vi "QMH_create.vi"(8 "error in (no error)":errorcluster) -> (0 "error out":errorcluster)   [LabVIEW 2021, in "Framework_lib.lvlib"]
uses:
  Framework_lib.lvlib
  framework_Qmessage.ctl
  QMH_notifier_payload.ctl
  QMH_producer_enum.ctl
  QMH_references.ctl
  QMH_references_enum.ctl
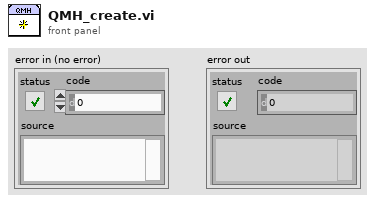
[diagram p1: front panel]
types:
  T1 = typedef "Framework_lib.lvlib/QMH_references_enum.ctl" = enum16{"--select Ref--", "Consumer_SUT", "Consumer_Annot", "Compute_Results"}
  T2 = typedef "Framework_lib.lvlib/QMH_references.ctl" = cluster{"Consumer_SUT":refnum<queue>, "Consumer_annotation":refnum<queue>, "compute_results":refnum<queue>, "Notifier":refnum<notifier>}
  T3 = typedef "Framework_lib.lvlib/QMH_notifier_payload.ctl" = cluster{"Message":T4, "Payload":variant}
  T4 = typedef "Framework_lib.lvlib/QMH_producer_enum.ctl" = enum16{"Idle", "Initialize", "Shutdown", "ERROR", "Stop", "Start", "Enqueue_frames"}
  T5 = typedef "Framework_lib.lvlib/framework_Qmessage.ctl" = cluster{"Message":string, "Payload":variant}
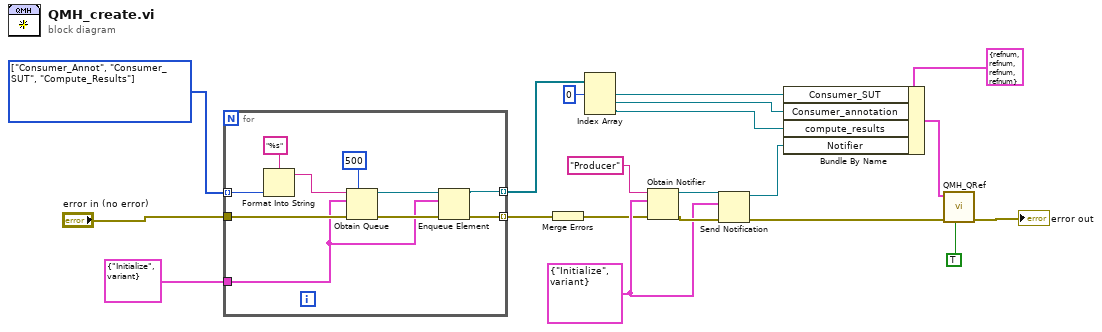
[diagram p0: block diagram]
diagram:
  w1 = T1[] [enum."Consumer_Annot", enum."Consumer_SUT", enum."Compute_Results"] items=["--select Ref--", "Consumer_SUT", "Consumer_Annot", "Compute_Results"] ("Array")
  w16 = T3 {"Message"=enum."Initialize", "Payload"=variant}
  n1 = for {
    tunnel: "error in (no error)" -> [w30]
    tunnel: w1 -> [w23] mode=indexing
    tunnel: T5 {"Message"="Initialize", "Payload"=variant} -> [w26]
    tunnel: [w25] -> w10 mode=indexing
    tunnel: [w24] -> w8 mode=indexing
    n2 = Format Into String(format string="%s", w23) -> (resulting string=w21:string)  [unwired: 2 in, 1 out]
    n3 = Obtain Queue(max queue size (-1, unlimited)=500, name (unnamed)=w21, element data type=w26, error in (no error)=w30) -> (queue out=w28:refnum<queue>, error out=w29:errorcluster)  [unwired: 1 in, 1 out]
    n4 = Enqueue Element(queue=w28, element=w26, error in (no error)=w29) -> (queue out=w24:refnum<queue>, error out=w25:errorcluster)  [unwired: 1 in, 1 out]
  }
  n5 = Merge Errors(w10) -> (w9:errorcluster)
  n6 = Index Array(array=w8, index #1=0 ("index")) -> (element #1=w6:refnum<queue>, element #2=w5:refnum<queue>, element #3=w2:refnum<queue>)  [unwired: 2 in]
  n7 = Obtain Notifier(name (unnamed)="Producer", notification data type=w16, error in (no error)=w9) -> (notifier out=w17:refnum<notifier>, error out=w19:errorcluster)  [unwired: 1 in, 1 out]
  n8 = Send Notification(notification=w16, notifier=w17, error in (no error)=w19) -> (notifier out=w4:refnum<notifier>, error out=w15:errorcluster)
  n9 = Bundle By Name(cluster=T2 {"Consumer_SUT"=refnum, "Consumer_annotation"=refnum, "compute_results"=refnum, "Notifier"=refnum} ("Cluster In"), "Consumer_SUT"=w6, "Consumer_annotation"=w5, "compute_results"=w2, "Notifier"=w4) -> (w12:T2)
  n10 = call "QMH_QRef.vi"("Get/Set (Get=F)"=TRUE ("Get (F)"), "error in (no error)"=w15, "Cluster In"=w12) -> ("error out"=→"error out":errorcluster)  [unwired: 6 in, 2 out]
